vi "Write bev.vi"(8 "error in (no error)":errorcluster, 10 "Beverage.lvclass":refnum<class "Beverage.lvclass">, 11 "Mocha in":refnum<class "Mocha.lvclass">) -> (0 "error out":errorcluster, 3 "Mocha out":refnum<class "Mocha.lvclass">)   [LabVIEW 2018, in "Mocha.lvclass"]
uses:
  Mocha.lvclass
  Beverage Class/Beverage.lvclass
  CondimentDecorator/CondimentDecorator.lvclass
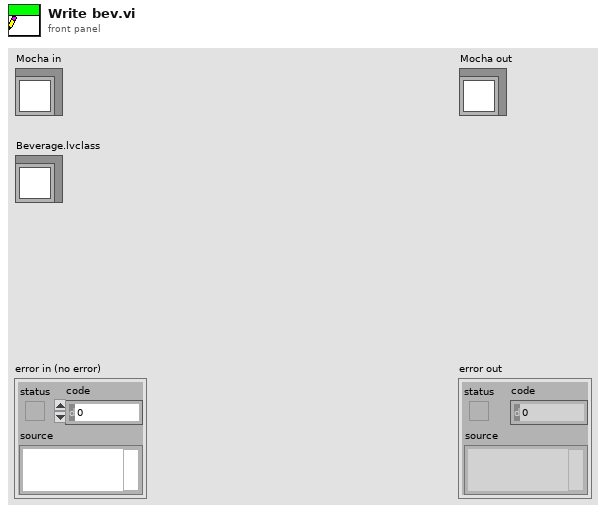
[diagram p1: front panel]
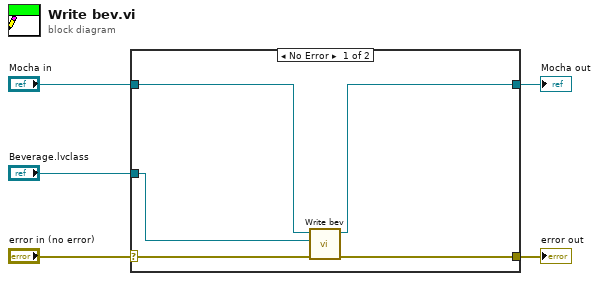
[diagram p0: block diagram]
diagram:
  n1 = case shown="No Error" "error in (no error)" {
    selector: "error in (no error)" -> [w10 w11]
    tunnel: [w9 w11] -> w4
    tunnel: [w7 w12] -> w2
    tunnel: "Mocha in" -> [w8 w12]
    tunnel: "Beverage.lvclass" -> [w6 _]
    frame No Error {
      n2 = call-parent "Write bev.vi"("error in (no error)"=w10, "Beverage.lvclass"=w6, "CondimentDecorator in"=w8) -> ("error out"=w9:errorcluster, "CondimentDecorator out"=w7:refnum<class "Mocha.lvclass">)  [unwired: 7 in]
    }
    frame Error {
    }
  }
  "error out" <- w4
  "Mocha out" <- w2
